vi "Write UpdateEvent.vi"(8 "error in (no error)":errorcluster, 10 "UpdateEvent":refnum<user-event>, 11 "VariableManager in":refnum<class "VariableManager.lvclass">) -> (0 "error out":errorcluster, 3 "VariableManager out":refnum<class "VariableManager.lvclass">)   [LabVIEW 2013, in "VariableManager.lvclass"]
uses:
  VariableManager.lvclass
  VariableManager.lvclass/VariableManager.ctl
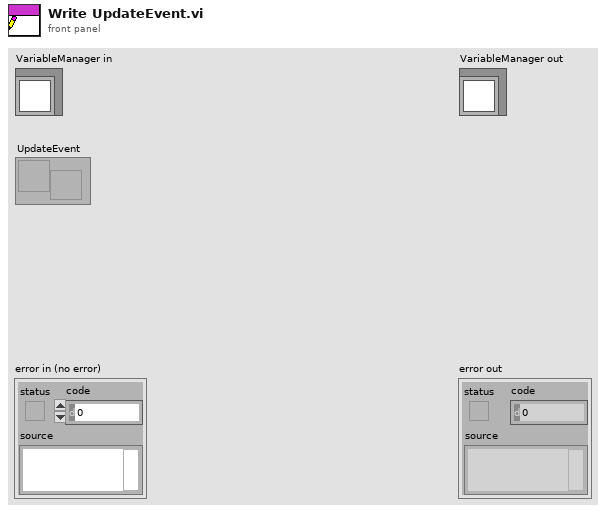
[diagram p1: front panel]
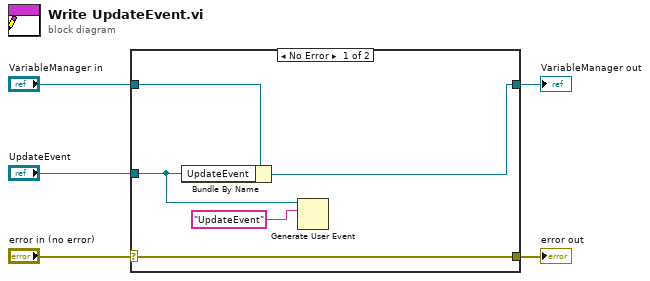
[diagram p0: block diagram]
diagram:
  n1 = case shown="No Error" "error in (no error)" {
    selector: "error in (no error)" -> [w10 w11]
    tunnel: [w10 w11] -> w4
    tunnel: [w8 w12] -> w2
    tunnel: "VariableManager in" -> [w9 w12]
    tunnel: "UpdateEvent" -> [w7 _]
    frame No Error {
      n2 = Bundle By Name(cluster=w9, "UpdateEvent"=w7) -> (w8:refnum<class "VariableManager.lvclass">)
      n3 = Generate User Event(user event=w7, event data cluster="UpdateEvent") -> ()  [unwired: 2 in, 2 out]
    }
    frame Error {
    }
  }
  "error out" <- w4
  "VariableManager out" <- w2
